vi "Swerve Open.vi"() -> ()   [LabVIEW 2017]
uses:
  <vilib>/Rock Robotics/WPI/ThirdParty/Phoenix-LabVIEW/Motor Controller/Controls/CTRE_Phoenix_MotorControl_FeedbackDevice.ctl
  <vilib>/Rock Robotics/WPI/ThirdParty/Phoenix-LabVIEW/Motor Controller/Controls/CTRE_Phoenix_MotorControl_VelocityMeasurementPeriod.ctl
  <vilib>/Rock Robotics/WPI/ThirdParty/Phoenix-LabVIEW/Motor Controller/Get/CTRE_Phoenix_MotorController_GetPulseWidthAll.vi
panel:
  in  "Offsets":dbl[](array[numeric])=[0.250198, -0.25301, 0.49432, 0.23414]
  in  "Constants":T1
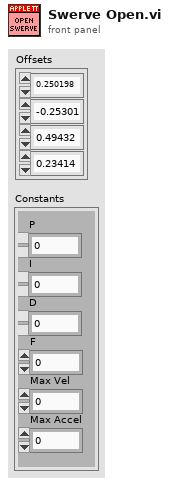
[diagram p1: front panel]
types:
  T1 = cluster{"P":dbl, "I":dbl, "D":dbl, "F":dbl, "Max Vel":dbl, "Max Accel":dbl}
  T2 = typedef "CTRE_Phoenix_MotorControl_VelocityMeasurementPeriod.ctl" = u16
  T3 = typedef "CTRE_Phoenix_MotorControl_FeedbackDevice.ctl" = i8
  T4 = typedef "WPI_MotorControlDeviceRef.ctl" = cluster{"DeviceStatus":errorcluster, "Type":T5, "PWM":cluster{"PWM Channel":T6, "DeadBand":T7}, "CAN":cluster{"Device Number":u8, "SetOutput VI Ref":variant, "GetOutput VI Ref":variant, "Enable VI Ref":variant, "Disable VI Ref":variant, "Data":variant}, "Invert":bool, "DIO PWM":cluster{"PWM \"Enable\" Channel":T6, "DIOChannel":T8, "PWM Rate":dbl}}
  T5 = typedef "WPI_MotorControlType.ctl" = enum16{"PWM", "CAN", "DIO PWM"}
  T6 = typedef "FPGA_DIOPWMChannel.ctl" = enum8{"PWM 0", "PWM 1", "PWM 2", "PWM 3", "PWM 4", "PWM 5", "PWM 6", "PWM 7", "PWM 8", "PWM 9", "PWM MXP 0", "PWM MXP 1", "PWM MXP 2", "PWM MXP 3", "PWM MXP 4", "PWM MXP 5", "PWM MXP 6", "PWM MXP 7", "PWM MXP 8", "PWM MXP 9", "Invalid"}
  T7 = typedef "WPI_PWMDeadband.ctl" = cluster{"Name":string, "maxPositivePwm":i32, "minPositivePwm":i32, "centerPwm":i32, "maxNegativePwm":i32, "minNegativePwm":i32, "angularRange":u16}
  T8 = typedef "FPGA_DIOChannel.ctl" = enum8{"DIO 0", "DIO 1", "DIO 2", "DIO 3", "DIO 4", "DIO 5", "DIO 6", "DIO 7", "DIO 8", "DIO 9", "DIO MXP 0", "DIO MXP 1", "DIO MXP 2", "DIO MXP 3", "DIO MXP 4", "DIO MXP 5", "DIO MXP 6", "DIO MXP 7", "DIO MXP 8", "DIO MXP 9", "DIO MXP 10", "DIO MXP 11", "DIO MXP 12", "DIO MXP 13", "DIO MXP 14", "DIO MXP 15", "SPI Port CS1", "SPI Port CS2", "SPI Port CS3", "SPI Port MISO", "SPI Port MOSI", "Invalid"}
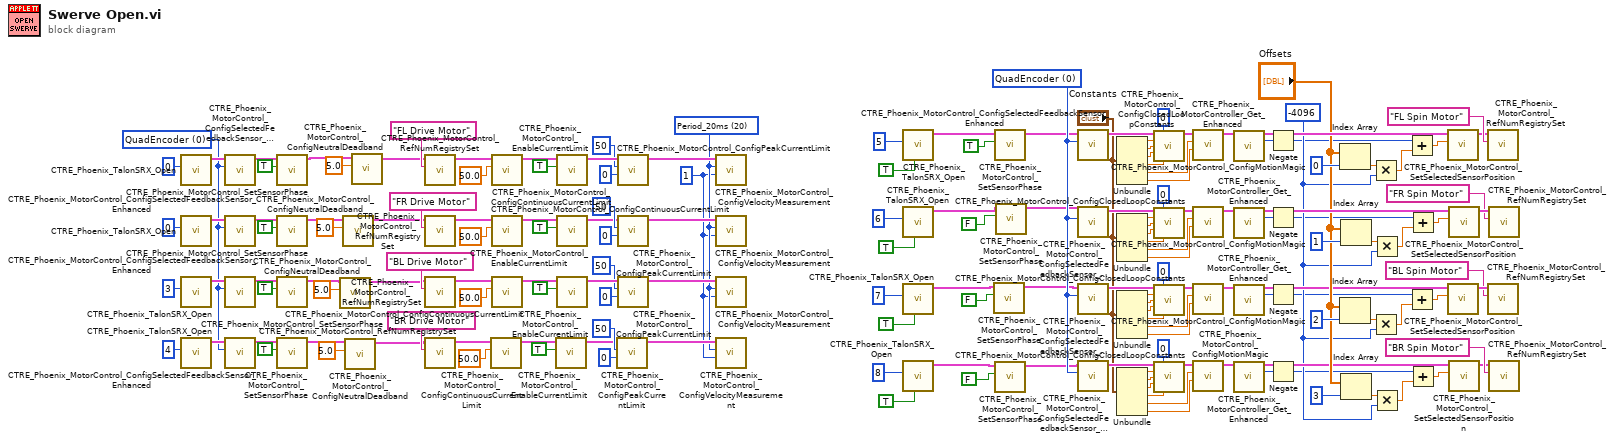
[diagram p0: block diagram]
diagram:
  w27 = T2 20 items=["Period_1ms"=1, "Period_2ms"=2, "Period_5ms"=5, "Period_10ms"=10, "Period_20ms"=20, "Period_25ms"=25, "Period_50ms"=50, "Period_100ms"=100] ("Velocity Measurement Period")
  w26 = 1 ("Peak Current (Amps)")
  w67 = T3 0 items=["None"=-1, "QuadEncoder"=0, "Analog"=2, "Tachometer"=4, "Pulse Width Encoded Position"=8, "Sensor Sum (S0 + S1)"=9, "Sensor Difference (D0 - D1)"=10, "Remote Source 0"=11, "Remote Source 1"=12, "Software Emulated"=15] ("Feedback Device")
  (unwired) u8 0 ("Device Number")
  (unwired) u8 0 ("Device Number")
  (unwired) u8 0 ("Device Number")
  (unwired) u8 0 ("Device Number")
  w82 = -4096 ("y")
  w13 = T3 0 items=["None"=-1, "QuadEncoder"=0, "Analog"=2, "Tachometer"=4, "Pulse Width Encoded Position"=8, "Sensor Sum (S0 + S1)"=9, "Sensor Difference (D0 - D1)"=10, "Remote Source 0"=11, "Remote Source 1"=12, "Software Emulated"=15] ("Feedback Device")
  n1 = call <vilib>:"CTRE_Phoenix_TalonSRX_Open.vi"("Device Number"=u8 1) -> ("CAN Talon SRX Ref"=w71:T4)  [unwired: 9 in, 1 out]
  n2 = call <vilib>:"CTRE_Phoenix_TalonSRX_Open.vi"("Device Number"=u8 2) -> ("CAN Talon SRX Ref"=w70:T4)  [unwired: 9 in, 1 out]
  n3 = call <vilib>:"CTRE_Phoenix_TalonSRX_Open.vi"("Device Number"=u8 3) -> ("CAN Talon SRX Ref"=w69:T4)  [unwired: 9 in, 1 out]
  n4 = call <vilib>:"CTRE_Phoenix_TalonSRX_Open.vi"("Device Number"=u8 4) -> ("CAN Talon SRX Ref"=w72:T4)  [unwired: 9 in, 1 out]
  n5 = call <vilib>:"CTRE_Phoenix_MotorControl_ConfigSelectedFeedbackSensor_Enhanced.vi"("Feedback Device"=w67, "PhoenixMotorControlDevRef"=w71) -> ("PhoenixMotorControlDevRef"=w68:T4)  [unwired: 8 in, 1 out]
  n6 = call <vilib>:"CTRE_Phoenix_MotorControl_ConfigSelectedFeedbackSensor_Enhanced.vi"("Feedback Device"=w67, "PhoenixMotorControlDevRef"=w70) -> ("PhoenixMotorControlDevRef"=w64:T4)  [unwired: 8 in, 1 out]
  n7 = call <vilib>:"CTRE_Phoenix_MotorControl_ConfigSelectedFeedbackSensor_Enhanced.vi"("Feedback Device"=w67, "PhoenixMotorControlDevRef"=w69) -> ("PhoenixMotorControlDevRef"=w65:T4)  [unwired: 8 in, 1 out]
  n8 = call <vilib>:"CTRE_Phoenix_MotorControl_ConfigSelectedFeedbackSensor_Enhanced.vi"("Feedback Device"=w67, "PhoenixMotorControlDevRef"=w72) -> ("PhoenixMotorControlDevRef"=w66:T4)  [unwired: 8 in, 1 out]
  n9 = call <vilib>:"CTRE_Phoenix_MotorControl_SetSensorPhase.vi"("PhaseSensor"=TRUE, "PhoenixMotorControlDevRef"=w68) -> ("PhoenixMotorControlDevRef"=w24:T4)  [unwired: 8 in, 1 out]
  n10 = call <vilib>:"CTRE_Phoenix_MotorControl_SetSensorPhase.vi"("PhaseSensor"=TRUE, "PhoenixMotorControlDevRef"=w64) -> ("PhoenixMotorControlDevRef"=w22:T4)  [unwired: 8 in, 1 out]
  n11 = call <vilib>:"CTRE_Phoenix_MotorControl_SetSensorPhase.vi"("PhaseSensor"=TRUE, "PhoenixMotorControlDevRef"=w65) -> ("PhoenixMotorControlDevRef"=w19:T4)  [unwired: 8 in, 1 out]
  n12 = call <vilib>:"CTRE_Phoenix_MotorControl_SetSensorPhase.vi"("PhaseSensor"=TRUE, "PhoenixMotorControlDevRef"=w66) -> ("PhoenixMotorControlDevRef"=w16:T4)  [unwired: 8 in, 1 out]
  n13 = call <vilib>:"CTRE_Phoenix_MotorControl_ConfigNeutralDeadband.vi"("Percent Deadband"=5.0, "PhoenixMotorControlDevRef"=w19) -> ("PhoenixMotorControlDevRef"=w18:T4)  [unwired: 8 in, 1 out]
  n14 = call <vilib>:"CTRE_Phoenix_MotorControl_ConfigNeutralDeadband.vi"("Percent Deadband"=5.0, "PhoenixMotorControlDevRef"=w22) -> ("PhoenixMotorControlDevRef"=w21:T4)  [unwired: 8 in, 1 out]
  n15 = call <vilib>:"CTRE_Phoenix_MotorControl_ConfigNeutralDeadband.vi"("Percent Deadband"=5.0, "PhoenixMotorControlDevRef"=w16) -> ("PhoenixMotorControlDevRef"=w15:T4)  [unwired: 8 in, 1 out]
  n16 = call <vilib>:"CTRE_Phoenix_MotorControl_ConfigNeutralDeadband.vi"("Percent Deadband"=5.0, "PhoenixMotorControlDevRef"=w24) -> ("PhoenixMotorControlDevRef"=w25:T4)  [unwired: 8 in, 1 out]
  n17 = call <vilib>:"CTRE_Phoenix_MotorControl_RefNumRegistrySet.vi"("refnum name"="FL Drive Motor", "PhoenixMotorControlDevRef"=w25) -> ("PhoenixMotorControlDevRef"=w34:T4)  [unwired: 8 in, 1 out]
  n18 = call <vilib>:"CTRE_Phoenix_MotorControl_RefNumRegistrySet.vi"("refnum name"="FR Drive Motor", "PhoenixMotorControlDevRef"=w21) -> ("PhoenixMotorControlDevRef"=w33:T4)  [unwired: 8 in, 1 out]
  n19 = call <vilib>:"CTRE_Phoenix_MotorControl_RefNumRegistrySet.vi"("refnum name"="BL Drive Motor", "PhoenixMotorControlDevRef"=w18) -> ("PhoenixMotorControlDevRef"=w32:T4)  [unwired: 8 in, 1 out]
  n20 = call <vilib>:"CTRE_Phoenix_MotorControl_RefNumRegistrySet.vi"("refnum name"="BR Drive Motor", "PhoenixMotorControlDevRef"=w15) -> ("PhoenixMotorControlDevRef"=w53:T4)  [unwired: 8 in, 1 out]
  n21 = call <vilib>:"CTRE_Phoenix_MotorControl_ConfigContinuousCurrentLimit.vi"("Continuous Current Limit (Amps)"=50.0, "PhoenixMotorControlDevRef"=w53) -> ("PhoenixMotorControlDevRef"=w58:T4)  [unwired: 8 in, 1 out]
  n22 = call <vilib>:"CTRE_Phoenix_MotorControl_ConfigContinuousCurrentLimit.vi"("Continuous Current Limit (Amps)"=50.0, "PhoenixMotorControlDevRef"=w34) -> ("PhoenixMotorControlDevRef"=w36:T4)  [unwired: 8 in, 1 out]
  n23 = call <vilib>:"CTRE_Phoenix_MotorControl_ConfigContinuousCurrentLimit.vi"("Continuous Current Limit (Amps)"=50.0, "PhoenixMotorControlDevRef"=w33) -> ("PhoenixMotorControlDevRef"=w45:T4)  [unwired: 8 in, 1 out]
  n24 = call <vilib>:"CTRE_Phoenix_MotorControl_ConfigContinuousCurrentLimit.vi"("Continuous Current Limit (Amps)"=50.0, "PhoenixMotorControlDevRef"=w32) -> ("PhoenixMotorControlDevRef"=w48:T4)  [unwired: 8 in, 1 out]
  n25 = call <vilib>:"CTRE_Phoenix_MotorControl_EnableCurrentLimit.vi"("Enable Current Limit?"=TRUE, "PhoenixMotorControlDevRef"=w58) -> ("PhoenixMotorControlDevRef"=w54:T4)  [unwired: 8 in, 1 out]
  n26 = call <vilib>:"CTRE_Phoenix_MotorControl_EnableCurrentLimit.vi"("Enable Current Limit?"=TRUE, "PhoenixMotorControlDevRef"=w36) -> ("PhoenixMotorControlDevRef"=w40:T4)  [unwired: 8 in, 1 out]
  n27 = call <vilib>:"CTRE_Phoenix_MotorControl_EnableCurrentLimit.vi"("Enable Current Limit?"=TRUE, "PhoenixMotorControlDevRef"=w45) -> ("PhoenixMotorControlDevRef"=w41:T4)  [unwired: 8 in, 1 out]
  n28 = call <vilib>:"CTRE_Phoenix_MotorControl_EnableCurrentLimit.vi"("Enable Current Limit?"=TRUE, "PhoenixMotorControlDevRef"=w48) -> ("PhoenixMotorControlDevRef"=w52:T4)  [unwired: 8 in, 1 out]
  n29 = call <vilib>:"CTRE_Phoenix_MotorControl_ConfigPeakCurrentLimit.vi"("Peak Current Maximum Duration (ms)"=0, "Peak Current (Amps)"=50, "PhoenixMotorControlDevRef"=w54) -> ("PhoenixMotorControlDevRef"=w31:T4)  [unwired: 7 in, 1 out]
  n30 = call <vilib>:"CTRE_Phoenix_MotorControl_ConfigPeakCurrentLimit.vi"("Peak Current Maximum Duration (ms)"=0, "Peak Current (Amps)"=50, "PhoenixMotorControlDevRef"=w40) -> ("PhoenixMotorControlDevRef"=w30:T4)  [unwired: 7 in, 1 out]
  n31 = call <vilib>:"CTRE_Phoenix_MotorControl_ConfigPeakCurrentLimit.vi"("Peak Current Maximum Duration (ms)"=0, "Peak Current (Amps)"=50, "PhoenixMotorControlDevRef"=w41) -> ("PhoenixMotorControlDevRef"=w29:T4)  [unwired: 7 in, 1 out]
  n32 = call <vilib>:"CTRE_Phoenix_MotorControl_ConfigPeakCurrentLimit.vi"("Peak Current Maximum Duration (ms)"=0, "Peak Current (Amps)"=50, "PhoenixMotorControlDevRef"=w52) -> ("PhoenixMotorControlDevRef"=w28:T4)  [unwired: 7 in, 1 out]
  n33 = call <vilib>:"CTRE_Phoenix_MotorControl_ConfigVelocityMeasurement.vi"("Window Size"=w26, "Velocity Measurement Period"=w27, "PhoenixMotorControlDevRef"=w30) -> ()  [unwired: 7 in, 2 out]
  n34 = call <vilib>:"CTRE_Phoenix_MotorControl_ConfigVelocityMeasurement.vi"("Window Size"=w26, "Velocity Measurement Period"=w27, "PhoenixMotorControlDevRef"=w29) -> ()  [unwired: 7 in, 2 out]
  n35 = call <vilib>:"CTRE_Phoenix_MotorControl_ConfigVelocityMeasurement.vi"("Window Size"=w26, "Velocity Measurement Period"=w27, "PhoenixMotorControlDevRef"=w28) -> ()  [unwired: 7 in, 2 out]
  n36 = call <vilib>:"CTRE_Phoenix_MotorControl_ConfigVelocityMeasurement.vi"("Window Size"=w26, "Velocity Measurement Period"=w27, "PhoenixMotorControlDevRef"=w31) -> ()  [unwired: 7 in, 2 out]
  n37 = call <vilib>:"CTRE_Phoenix_TalonSRX_Open.vi"("Invert"=TRUE, "Device Number"=u8 5) -> ("CAN Talon SRX Ref"=w12:T4)  [unwired: 8 in, 1 out]
  n38 = call <vilib>:"CTRE_Phoenix_TalonSRX_Open.vi"("Invert"=TRUE, "Device Number"=u8 6) -> ("CAN Talon SRX Ref"=w10:T4)  [unwired: 8 in, 1 out]
  n39 = call <vilib>:"CTRE_Phoenix_TalonSRX_Open.vi"("Invert"=TRUE, "Device Number"=u8 7) -> ("CAN Talon SRX Ref"=w6:T4)  [unwired: 8 in, 1 out]
  n40 = call <vilib>:"CTRE_Phoenix_TalonSRX_Open.vi"("Invert"=TRUE, "Device Number"=u8 8) -> ("CAN Talon SRX Ref"=w2:T4)  [unwired: 8 in, 1 out]
  n41 = call <vilib>:"CTRE_Phoenix_MotorControl_SetSensorPhase.vi"("PhaseSensor"=FALSE, "PhoenixMotorControlDevRef"=w6) -> ("PhoenixMotorControlDevRef"=w5:T4)  [unwired: 8 in, 1 out]
  n42 = call <vilib>:"CTRE_Phoenix_MotorControl_SetSensorPhase.vi"("PhaseSensor"=TRUE, "PhoenixMotorControlDevRef"=w12) -> ("PhoenixMotorControlDevRef"=w11:T4)  [unwired: 8 in, 1 out]
  n43 = call <vilib>:"CTRE_Phoenix_MotorControl_SetSensorPhase.vi"("PhaseSensor"=FALSE, "PhoenixMotorControlDevRef"=w2) -> ("PhoenixMotorControlDevRef"=w1:T4)  [unwired: 8 in, 1 out]
  n44 = call <vilib>:"CTRE_Phoenix_MotorControl_SetSensorPhase.vi"("PhaseSensor"=FALSE, "PhoenixMotorControlDevRef"=w10) -> ("PhoenixMotorControlDevRef"=w9:T4)  [unwired: 8 in, 1 out]
  n45 = call <vilib>:"CTRE_Phoenix_MotorControl_ConfigSelectedFeedbackSensor_Enhanced.vi"("Feedback Device"=w13, "PhoenixMotorControlDevRef"=w11) -> ("PhoenixMotorControlDevRef"=w165:T4)  [unwired: 8 in, 1 out]
  n46 = call <vilib>:"CTRE_Phoenix_MotorControl_ConfigSelectedFeedbackSensor_Enhanced.vi"("Feedback Device"=w13, "PhoenixMotorControlDevRef"=w9) -> ("PhoenixMotorControlDevRef"=w152:T4)  [unwired: 8 in, 1 out]
  n47 = call <vilib>:"CTRE_Phoenix_MotorControl_ConfigSelectedFeedbackSensor_Enhanced.vi"("Feedback Device"=w13, "PhoenixMotorControlDevRef"=w5) -> ("PhoenixMotorControlDevRef"=w135:T4)  [unwired: 8 in, 1 out]
  n48 = call <vilib>:"CTRE_Phoenix_MotorControl_ConfigSelectedFeedbackSensor_Enhanced.vi"("Feedback Device"=w13, "PhoenixMotorControlDevRef"=w1) -> ("PhoenixMotorControlDevRef"=w148:T4)  [unwired: 8 in, 1 out]
  n49 = Unbundle("Constants") -> ("P"=w164:dbl, "I"=w163:dbl, "D"=w162:dbl, "F"=w161:dbl, "Max Vel"=w160:dbl, "Max Accel"=w159:dbl)
  n50 = Unbundle("Constants") -> ("P"=w153:dbl, "I"=w154:dbl, "D"=w155:dbl, "F"=w156:dbl, "Max Vel"=w157:dbl, "Max Accel"=w158:dbl)
  n51 = Unbundle("Constants") -> ("P"=w136:dbl, "I"=w137:dbl, "D"=w138:dbl, "F"=w139:dbl, "Max Vel"=w140:dbl, "Max Accel"=w141:dbl)
  n52 = Unbundle("Constants") -> ("P"=w147:dbl, "I"=w146:dbl, "D"=w145:dbl, "F"=w144:dbl, "Max Vel"=w143:dbl, "Max Accel"=w142:dbl)
  n53 = call <vilib>:"CTRE_Phoenix_MotorControl_ConfigClosedLoopConstants.vi"("PhoenixMotorControlDevRef"=w165, "slotIdx"=0, "P"=w164, "I"=w163, "D"=w162, "F"=w161) -> ("PhoenixMotorControlDevRef"=w166:T4)  [unwired: 8 in, 1 out]
  n54 = call <vilib>:"CTRE_Phoenix_MotorControl_ConfigClosedLoopConstants.vi"("PhoenixMotorControlDevRef"=w152, "slotIdx"=0, "P"=w153, "I"=w154, "D"=w155, "F"=w156) -> ("PhoenixMotorControlDevRef"=w151:T4)  [unwired: 8 in, 1 out]
  n55 = call <vilib>:"CTRE_Phoenix_MotorControl_ConfigClosedLoopConstants.vi"("PhoenixMotorControlDevRef"=w135, "slotIdx"=0, "P"=w136, "I"=w137, "D"=w138, "F"=w139) -> ("PhoenixMotorControlDevRef"=w134:T4)  [unwired: 8 in, 1 out]
  n56 = call <vilib>:"CTRE_Phoenix_MotorControl_ConfigClosedLoopConstants.vi"("PhoenixMotorControlDevRef"=w148, "slotIdx"=0, "P"=w147, "I"=w146, "D"=w145, "F"=w144) -> ("PhoenixMotorControlDevRef"=w149:T4)  [unwired: 8 in, 1 out]
  n57 = call <vilib>:"CTRE_Phoenix_MotorControl_ConfigMotionMagic.vi"("Acceleration"=w159, "Cruise Velocity"=w160, "PhoenixMotorControlDevRef"=w166) -> ("PhoenixMotorControlDevRef"=w167:T4)  [unwired: 7 in, 1 out]
  n58 = call <vilib>:"CTRE_Phoenix_MotorControl_ConfigMotionMagic.vi"("Acceleration"=w158, "Cruise Velocity"=w157, "PhoenixMotorControlDevRef"=w151) -> ("PhoenixMotorControlDevRef"=w150:T4)  [unwired: 7 in, 1 out]
  n59 = call <vilib>:"CTRE_Phoenix_MotorControl_ConfigMotionMagic.vi"("Acceleration"=w141, "Cruise Velocity"=w140, "PhoenixMotorControlDevRef"=w134) -> ("PhoenixMotorControlDevRef"=w133:T4)  [unwired: 7 in, 1 out]
  n60 = call <vilib>:"CTRE_Phoenix_MotorControl_ConfigMotionMagic.vi"("Acceleration"=w142, "Cruise Velocity"=w143, "PhoenixMotorControlDevRef"=w149) -> ("PhoenixMotorControlDevRef"=w77:T4)  [unwired: 7 in, 1 out]
  n61 = call-poly <vilib>:"CTRE_Phoenix_MotorController_Get_Enhanced.vi"("PhoenixMotorControlDevRef"=w167) -> ("PhoenixMotorControlDevRef"=w101:T4, "Pulse Width Position"=w100:i32)  [unwired: 9 in, 4 out]
  n62 = call-poly <vilib>:"CTRE_Phoenix_MotorController_Get_Enhanced.vi"("PhoenixMotorControlDevRef"=w150) -> ("PhoenixMotorControlDevRef"=w110:T4, "Pulse Width Position"=w109:i32)  [unwired: 9 in, 4 out]
  n63 = call-poly <vilib>:"CTRE_Phoenix_MotorController_Get_Enhanced.vi"("PhoenixMotorControlDevRef"=w133) -> ("PhoenixMotorControlDevRef"=w86:T4, "Pulse Width Position"=w85:i32)  [unwired: 9 in, 4 out]
  n64 = call-poly <vilib>:"CTRE_Phoenix_MotorController_Get_Enhanced.vi"("PhoenixMotorControlDevRef"=w77) -> ("PhoenixMotorControlDevRef"=w84:T4, "Pulse Width Position"=w83:i32)  [unwired: 9 in, 4 out]
  n65 = Negate(x=w100) -> (-x=w76:i32)
  n66 = Negate(x=w109) -> (-x=w75:i32)
  n67 = Negate(x=w85) -> (-x=w74:i32)
  n68 = Negate(x=w83) -> (-x=w73:i32)
  n69 = Index Array(array="Offsets", index=0) -> (element=w103:dbl)
  n70 = Index Array(array="Offsets", index=2) -> (element=w98:dbl)
  n71 = Index Array(array="Offsets", index=1) -> (element=w115:dbl)
  n72 = Index Array(array="Offsets", index=3) -> (element=w88:dbl)
  n73 = Multiply(x=w103, y=w82) -> (x*y=w105:dbl)
  n74 = Multiply(x=w98, y=w82) -> (x*y=w96:dbl)
  n75 = Multiply(x=w115, y=w82) -> (x*y=w113:dbl)
  n76 = Multiply(x=w88, y=w82) -> (x*y=w90:dbl)
  n77 = Add(x=w76, y=w105) -> (x+y=w104:dbl)
  n78 = Add(x=w74, y=w96) -> (x+y=w97:dbl)
  n79 = Add(x=w75, y=w113) -> (x+y=w114:dbl)
  n80 = Add(x=w73, y=w90) -> (x+y=w89:dbl)
  n81 = call <vilib>:"CTRE_Phoenix_MotorControl_SetSelectedSensorPosition.vi"("New Sensor Position"=w104, "PhoenixMotorControlDevRef"=w101) -> ("PhoenixMotorControlDevRef"=w106:T4)  [unwired: 8 in, 1 out]
  n82 = call <vilib>:"CTRE_Phoenix_MotorControl_SetSelectedSensorPosition.vi"("New Sensor Position"=w97, "PhoenixMotorControlDevRef"=w86) -> ("PhoenixMotorControlDevRef"=w95:T4)  [unwired: 8 in, 1 out]
  n83 = call <vilib>:"CTRE_Phoenix_MotorControl_SetSelectedSensorPosition.vi"("New Sensor Position"=w114, "PhoenixMotorControlDevRef"=w110) -> ("PhoenixMotorControlDevRef"=w111:T4)  [unwired: 8 in, 1 out]
  n84 = call <vilib>:"CTRE_Phoenix_MotorControl_SetSelectedSensorPosition.vi"("New Sensor Position"=w89, "PhoenixMotorControlDevRef"=w84) -> ("PhoenixMotorControlDevRef"=w92:T4)  [unwired: 8 in, 1 out]
  n85 = call <vilib>:"CTRE_Phoenix_MotorControl_RefNumRegistrySet.vi"("refnum name"="FL Spin Motor", "PhoenixMotorControlDevRef"=w106) -> ()  [unwired: 8 in, 2 out]
  n86 = call <vilib>:"CTRE_Phoenix_MotorControl_RefNumRegistrySet.vi"("refnum name"="BL Spin Motor", "PhoenixMotorControlDevRef"=w95) -> ()  [unwired: 8 in, 2 out]
  n87 = call <vilib>:"CTRE_Phoenix_MotorControl_RefNumRegistrySet.vi"("refnum name"="FR Spin Motor", "PhoenixMotorControlDevRef"=w111) -> ()  [unwired: 8 in, 2 out]
  n88 = call <vilib>:"CTRE_Phoenix_MotorControl_RefNumRegistrySet.vi"("refnum name"="BR Spin Motor", "PhoenixMotorControlDevRef"=w92) -> ()  [unwired: 8 in, 2 out]
